vi "Teleop Drivetrain Control.vi"(9 "D-Pad":T1, 10 "Button Cluster":T2, 11 "Axes":T3) -> ()   [LabVIEW 2017]
uses:
  Common Code/Gamepads/Axes Cluster.ctl
  Common Code/Gamepads/Button Cluster.ctl
  Common Code/Gamepads/D-Pad.ctl
  Common Code/Drivetrain Mode.ctl
  Common Code/Utilities/Change Detect.vi
  Common Code/Utilities/Change Detect Boolean.vi
  Robot Global Data.vi
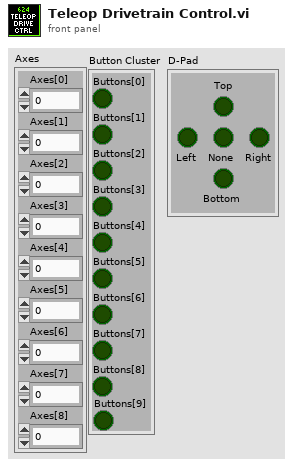
[diagram p1: front panel]
types:
  T1 = typedef "D-Pad.ctl" = cluster{"Top":bool, "Bottom":bool, "None":bool, "Right":bool, "Left":bool}
  T2 = typedef "Button Cluster.ctl" = cluster{"Buttons[0]":bool, "Buttons[1]":bool, "Buttons[2]":bool, "Buttons[3]":bool, "Buttons[4]":bool, "Buttons[5]":bool, "Buttons[6]":bool, "Buttons[7]":bool, "Buttons[8]":bool, "Buttons[9]":bool}
  T3 = typedef "Axes Cluster.ctl" = cluster{"Axes[0]":dbl, "Axes[1]":dbl, "Axes[2]":dbl, "Axes[3]":dbl, "Axes[4]":dbl, "Axes[5]":dbl, "Axes[6]":dbl, "Axes[7]":dbl, "Axes[8]":dbl}
  T4 = typedef "Drivetrain Mode.ctl" = enum16{"Manual", "Gyro Steer", "PID Drive", "Distance Drive", "Autonomous"}
  T5 = typedef "Dashboard Control Data.ctl" = cluster{"Drivetrain Settings Cluster":T6, "Intake Presets":T8, "Elevator Settings Cluster":T9, "Drivetrain Encoder Values":T11, "Auton Chooser":T12}
  T6 = typedef "Drivetrain Settings Cluster.ctl" = cluster{"Gyro Steer PID Gains":T7, "Distance Drive PID Gains":T7, "Drive Tolerance":dbl, "Gyro Tolerance":dbl, "Gyro Output":dbl, "Distance Output":dbl, "Y Power Multiplier":dbl, "Turn Power Multiplier":dbl, "Creep Rate":dbl, "Constant Power":bool, "DT Mode Modifier":enum16{"None, Default", "Cube", "Square"}, "Left Encoder Tick Constant":dbl, "Right Encoder Tick Constant":dbl, "Shift Speed":dbl}
  T7 = typedef "PID Gains Cluster.ctl" = cluster{"Integral Time":dbl, "Proportional Gain":dbl, "Derivative Time":dbl}
  T8 = typedef "Intake Presets.ctl" = cluster{"Idle Angle":dbl, "Mid Angle":dbl, "Low Angle":dbl, "Outtake Power":dbl, "Intake Power":dbl, "Unstuck":dbl, "Angle Tolerance":dbl, "Max Angle":dbl, "Max Current":dbl, "Current Trip Time":dbl, "Reset Encoder?":bool, "Encoder Scale":dbl, "PID gains":cluster{"proportional gain (Kc)":dbl, "integral time (Ti, min)":dbl, "derivative time (Td, min)":dbl}, "output range":cluster{"output high":dbl, "output low":dbl}}
  T9 = typedef "Elevator Settings Cluster.ctl" = cluster{"Ground Height":dbl, "Switch Height":dbl, "Scale High Height ":dbl, "Scale Low Height":dbl, "Elevator PID Gains":T10, "Elevator Tolerance":dbl, "Reset Encoders":bool, "Encoder Scale":dbl, "Max Height":dbl, "Mid Height":dbl, "output range":cluster{"output high":dbl, "output low":dbl}, "Slow Down Tolerance":dbl}
  T10 = typedef "PID Gains.ctl" = cluster{"proportional gain (Kc)":dbl, "integral time (Ti, min)":dbl, "derivative time (Td, min)":dbl}
  T11 = typedef "DT Encoder Values.ctl" = cluster{"Left Encoder":cluster{"Distance":dbl, "Speed":dbl, "Tick":dbl}, "Right Encoder":cluster{"Distance":dbl, "Speed":dbl, "Tick":dbl}}
  T12 = typedef "Auton Chooser.ctl" = cluster{"Left":bool, "Center":bool, "Right":bool, "Scale":bool, "Both":bool, "Switch":bool, "Near":bool, "Far":bool}
  T13 = typedef "Drivetrain Status Cluster.ctl" = cluster{"Throttle (Y)":dbl, "Steer (X)":dbl, "Drivetrain Mode":T4, "Brake?":bool, "Distance Drive Complete?":bool, "PID Drive Complete?":bool, "Creep Mode?":bool, "Gyro Steer Complete?":bool, "Gyro":dbl, "X Max Output":dbl, "X Min Output":dbl, "Y Max Output ":dbl, "Y Min Output":dbl, "Heading Target":dbl, "Distance Target":dbl, "2nd Gear":bool, "Drivetrain Encoder Values":T11}
  T14 = typedef "Drivetrain Command Cluster.ctl" = cluster{"Y Power":dbl, "Turn Power":dbl, "Drivetrain Mode":T4, "2nd Gear":bool, "Y Min Output":dbl, "Y Max Output":dbl, "X Min Output":dbl, "X Max Output":dbl, "Heading Target":dbl, "Distance Target":dbl, "Brake?":bool, "Zero Gyro":bool}
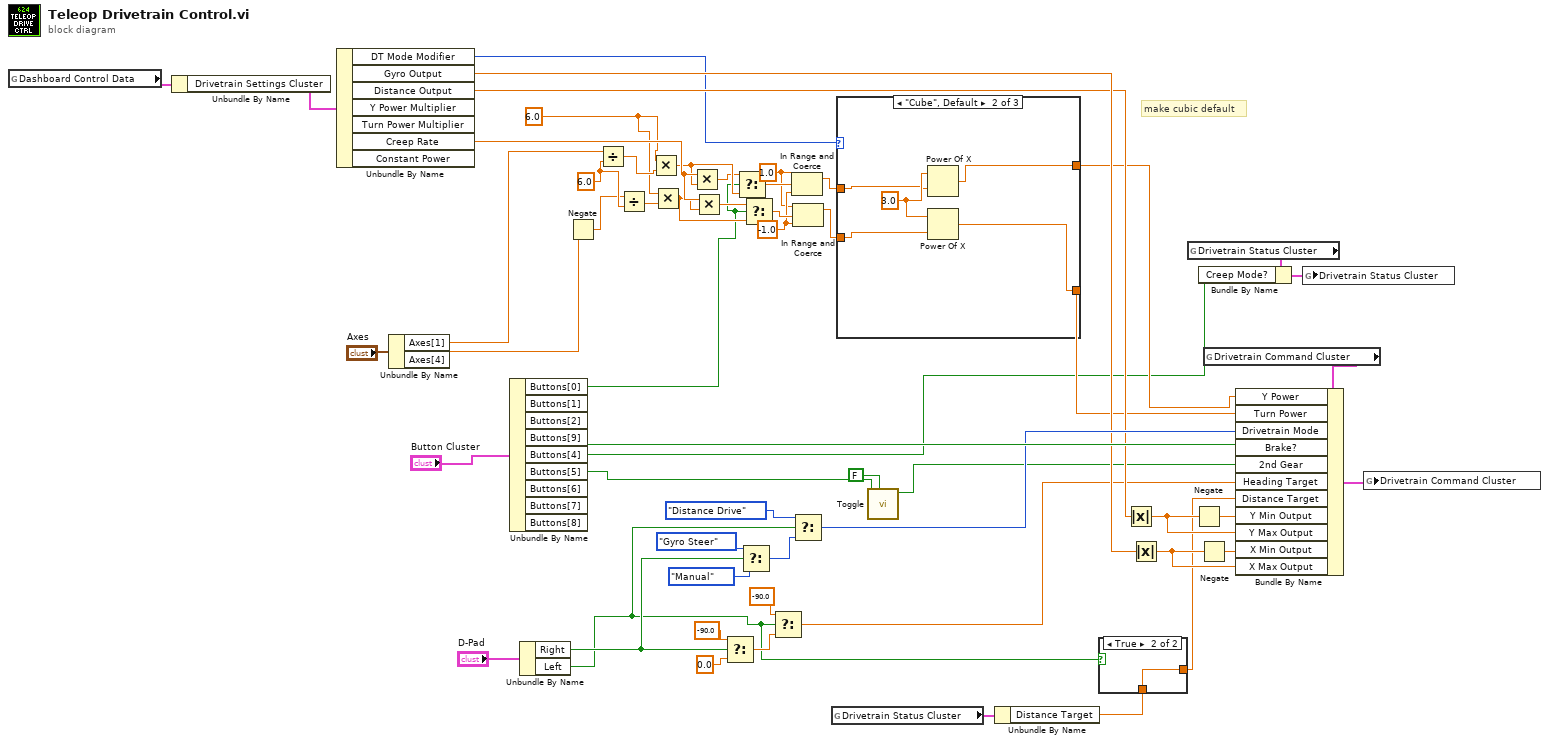
[diagram p0: block diagram]
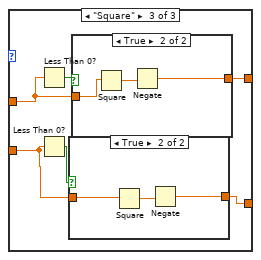
[diagram p3: hidden frame]
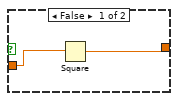
[diagram p4: hidden frame]
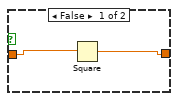
[diagram p5: hidden frame]
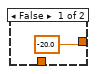
[diagram p6: hidden frame]
diagram:
  w2 = 6.0
  w9 = -1.0
  w8 = 1.0
  w23 = 6.0
  # "make cubic default"
  n1 = global read "Robot Global Data.vi" "Dashboard Control Data"() -> (w34:T5)
  n2 = Unbundle By Name(w34) -> ("Drivetrain Settings Cluster"=w33:T6)
  n3 = Unbundle By Name(w33) -> ("DT Mode Modifier"=w18:enum16{"None, Default", "Cube", "Square"}, "Gyro Output"=w31:dbl, "Distance Output"=w27:dbl, "Creep Rate"=w17:dbl)  [unwired: 3 out]
  n4 = Unbundle By Name("Axes") -> ("Axes[1]"=w21:dbl, "Axes[4]"=w3:dbl)
  n5 = Unbundle By Name("Button Cluster") -> ("Buttons[0]"=w12:bool, "Buttons[9]"=w48:bool, "Buttons[4]"=w1:bool, "Buttons[5]"=w36:bool)  [unwired: 5 out]
  n6 = Unbundle By Name("D-Pad") -> ("Right"=w41:bool, "Left"=w37:bool)
  n7 = Negate(x=w3) -> (-x=w22:dbl)
  n8 = Divide(x=w21, y=w23) -> (x/y=w19:dbl)
  n9 = Divide(x=w22, y=w23) -> (x/y=w20:dbl)
  n10 = Multiply(x=w2, y=w19) -> (x*y=w16:dbl)
  n11 = Multiply(x=w2, y=w20) -> (x*y=w13:dbl)
  n12 = Multiply(x=w17, y=w16) -> (x*y=w15:dbl)
  n13 = Multiply(x=w17, y=w13) -> (x*y=w14:dbl)
  n14 = Select(t=-90.0, s=w41, f=0.0) -> (s? t:f=w51:dbl)
  n15 = Select(t=w15, s=w12, f=w16) -> (s? t:f=w11:dbl)
  n16 = Select(t=Drivetrain_Mode."Gyro Steer" ("Drivetrain Mode"), s=w41, f=Drivetrain_Mode."Manual" ("Drivetrain Mode")) -> (s? t:f=w40:T4)
  n17 = Select(t=w14, s=w12, f=w13) -> (s? t:f=w10:dbl)
  n18 = Select(t=-90.0, s=w37, f=w51) -> (s? t:f=w25:dbl)
  n19 = In Range and Coerce(upper limit=w8, x=w11, lower limit=w9) -> (coerced(x)=w7:dbl)  [unwired: 1 out]
  n20 = In Range and Coerce(upper limit=w8, x=w10, lower limit=w9) -> (coerced(x)=w6:dbl)  [unwired: 1 out]
  n21 = Select(t=Drivetrain_Mode."Distance Drive" ("Drivetrain Mode"), s=w37, f=w40) -> (s? t:f=w38:T4)
  n22 = global read "Robot Global Data.vi" "Drivetrain Status Cluster"() -> (w47:T13)
  n23 = case shown="\"Cube\", Default" w18 {
    tunnel: w7 -> [w59 w63 w68]
    tunnel: w6 -> [w58 w62 w65]
    tunnel: [w59 w61 w67] -> w5
    tunnel: [w58 w60 w66] -> w4
    frame "None, Default" {
    }
    frame "Cube", Default {
      w64 = 3.0
      n24 = Power Of X(1:w63, 2:w64) -> (0:w61:dbl)
      n25 = Power Of X(1:w62, 2:w64) -> (0:w60:dbl)
    }
    frame "Square" {
      n26 = Less Than 0?(x=w68) -> (x < 0?=w69:bool)
      n27 = Less Than 0?(x=w65) -> (x < 0?=w70:bool)
      n28 = case shown="True" w70 {
        tunnel: [w76 w79] -> w66
        tunnel: w65 -> [w77 w78]
        frame False {
          n29 = Square(x=w77) -> (x^2=w76:dbl)
        }
        frame True {
          n30 = Square(x=w78) -> (x^2=w80:dbl)
          n31 = Negate(x=w80) -> (-x=w79:dbl)
        }
      }
      n32 = case shown="True" w69 {
        tunnel: w68 -> [w72 w74]
        tunnel: [w71 w73] -> w67
        frame False {
          n33 = Square(x=w72) -> (x^2=w71:dbl)
        }
        frame True {
          n34 = Square(x=w74) -> (x^2=w75:dbl)
          n35 = Negate(x=w75) -> (-x=w73:dbl)
        }
      }
    }
  }
  n36 = call "Toggle.vi"("Initial Value"=FALSE, "In"=w36) -> ("Toggled"=w26:bool)  [unwired: 9 in]
  n37 = Unbundle By Name(w47) -> ("Distance Target"=w46:dbl)
  n38 = case shown="True" w37 {
    tunnel: [-20.0 w82] -> w24
    tunnel: w46 -> [_ w82]
    frame False {
    }
    frame True {
    }
  }
  n39 = Absolute Value(x=w27) -> (abs(x)=w28:dbl)
  n40 = Absolute Value(x=w31) -> (abs(x)=w30:dbl)
  n41 = global read "Robot Global Data.vi" "Drivetrain Status Cluster"() -> (w45:T13)
  n42 = Negate(x=w28) -> (-x=w29:dbl)
  n43 = Bundle By Name(cluster=w45, "Creep Mode?"=w1) -> (w44:T13)
  n44 = Negate(x=w30) -> (-x=w32:dbl)
  n45 = global read "Robot Global Data.vi" "Drivetrain Command Cluster"() -> (w50:T14)
  n46 = Bundle By Name(cluster=w50, "Y Power"=w5, "Turn Power"=w4, "Drivetrain Mode"=w38, "Brake?"=w48, "2nd Gear"=w26, "Heading Target"=w25, "Distance Target"=w24, "Y Min Output"=w29, "Y Max Output"=w28, "X Min Output"=w32, "X Max Output"=w30) -> (w49:T14)
  n47 = global write "Robot Global Data.vi" "Drivetrain Status Cluster"(w44) -> ()
  n48 = global write "Robot Global Data.vi" "Drivetrain Command Cluster"(w49) -> ()
